vi "String to first letter lowercase(SubVI).vi"(11 "Couleur carré":string[](array[string])) -> (3 "String":string)   [LabVIEW 2019]
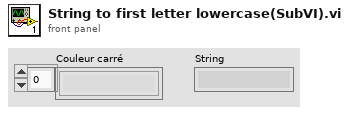
[diagram p1: front panel]
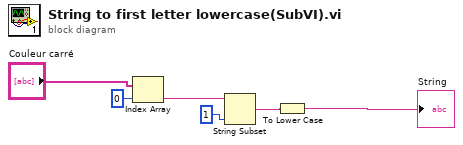
[diagram p0: block diagram]
diagram:
  n1 = Index Array(array="Couleur carré", index=0) -> (element=w4:string)
  n2 = String Subset(string=w4, length (rest)=1 ("length (rest)")) -> (substring=w5:string)  [unwired: 1 in]
  n3 = To Lower Case(string=w5) -> (all lower case string=→"String":string)
